vi "ScriptNotificationExample.vi"   [LabVIEW 2011]
uses:
  Main/GlobalVariables.vi
panel:
  # "Try running an experiment script with \"test event 123\" while this module is running"
types:
  T1 = typedef "QueueListType.ctl" = cluster{"Motor In":refnum<queue>, "User Interface Image View":refnum<queue>, "User Interface Camera Control":refnum<queue>, "User Interface Event Notifier":refnum<notifier>, "Initialized?":bool, "Experiment Script Event Notifier":refnum<notifier>}
  T2 = typedef "ScriptEventType.ctl" = cluster{"Text":string, "Is Simulation?":bool}
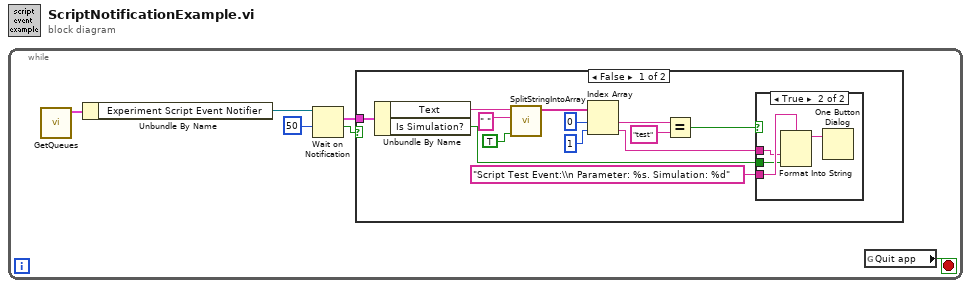
[diagram p0: block diagram]
diagram:
  n1 = while {
    stop <- w6 stop-if-true
    n2 = call "GetQueues.vi"() -> ("Queue List"=w5:T1)  [unwired: 10 in, 1 out]
    n3 = Unbundle By Name(w5) -> ("Experiment Script Event Notifier"=w4:refnum<notifier>)
    n4 = Wait on Notification(notifier=w4, timeout in ms (-1)=50) -> (notification=w2:T2, timed out?=w1:bool)  [unwired: 2 in, 2 out]
    n5 = case shown="False" w1 {
      tunnel: w2 -> [w19 _]
      frame False {
        n6 = Unbundle By Name(w19) -> ("Text"=w18:string, "Is Simulation?"=w7:bool)
        n7 = call "SplitStringIntoArray.vi"("remove empty entries? (F)"=TRUE, "seperators"=" ", "text"=w18) -> ("result"=w15:string[])  [unwired: 7 in, 1 out]
        n8 = Index Array(array=w15, index #1=0 ("index"), index #2=1 ("index")) -> (element #1=w11:string, element #2=w8:string)
        n9 = Equal?(x=w11, y="test") -> (x = y?=w9:bool)
        n10 = case shown="True" w9 {
          tunnel: "Script Test Event:\\n Parameter: %s. Simulation: %d" ("format string") -> [_ w23]
          tunnel: w8 -> [_ w21]
          tunnel: w7 -> [_ w20]
          frame False {
          }
          frame True {
            n11 = Format Into String(format string=w23, w21, w20) -> (resulting string=w22:string)  [unwired: 2 in, 1 out]
            n12 = One Button Dialog(message=w22) -> ()  [unwired: 1 in, 1 out]
          }
        }
      }
      frame True {
      }
    }
    n13 = global read "GlobalVariables.vi" "Quit app"() -> (w6:bool)
  }
